vi "VI, Set Window Size.vi"(4 "h (100)":i16=100, 5 "w (100)":i16=100, 6 "error in":errorcluster, 9 "VI ref":refnum<vi>) -> (0 "error out":errorcluster, 3 "VI ref dup":refnum<vi>)   [LabVIEW 2010]
doc: "This function sets the front panel window size in screen coordinates. The front panel window includes the interior region, scroll bars, title bar, menu bar, and toolbar. Screen coordinates are in pixel units and refer to the computer monitor screen (rather than an open window).\n\nYou can set this property only for VIs with open front panels."
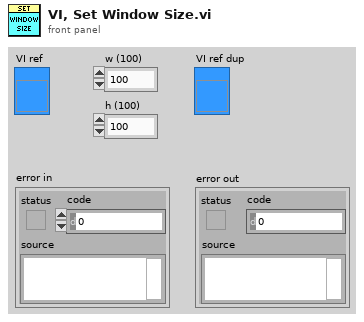
[diagram p1: front panel]
types:
  T1 = typedef "LVRectTypeDef.ctl" = cluster{"left":i16, "top":i16, "right":i16, "bottom":i16}
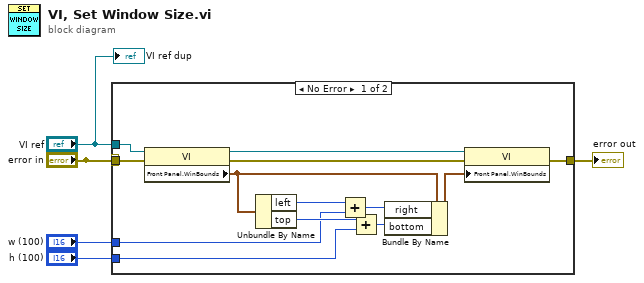
[diagram p0: block diagram]
diagram:
  n1 = case shown="No Error" "error in" {
    selector: "error in" -> [w18 w19]
    tunnel: [w15 w19] -> w5
    tunnel: "VI ref" -> [w17 _]
    tunnel: "error in" -> [_ _]
    tunnel: "h (100)" -> [w6 _]
    tunnel: "w (100)" -> [w7 _]
    frame No Error {
      n2 = property class="VI"(reference=w17, error in=w18) -> (reference out=w14:refnum<vi>, error out=w16:errorcluster, "Front Panel.WinBounds"=w12:T1)
      n3 = Unbundle By Name(w12) -> ("left"=w11:i16, "top"=w9:i16)
      n4 = Add(x=w11, y=w7) -> (x+y=w10:i16)
      n5 = Add(x=w9, y=w6) -> (x+y=w8:i16)
      n6 = Bundle By Name(cluster=w12, "right"=w10, "bottom"=w8) -> (w13:T1)
      n7 = property class="VI"(reference=w14, error in=w16, "Front Panel.WinBounds"=w13) -> (error out=w15:errorcluster)  [unwired: 1 out]
    }
    frame Error {
    }
  }
  "error out" <- w5
  "VI ref dup" <- "VI ref"
